vi "Main_Function_Motion Control.vi"(7 "Motion_Action":T3, 8 "Error In":errorcluster, 10 "Paremeter":T1={"Scan speed"=1, "Power"=0, "Angle"=0.0, "X"=0, "X"=0, "Xc"=0} {"Power" items=["Abs"=2, "Rel"=3]; "Scan speed" items=["X"=1, "Y"=2, "Z"=3, "Rotation"=4]}, 11 "VISA In":refnum<visa-resource-name>) -> (0 "Error Out":errorcluster, 2 "Response":string, 3 "VISA Out":refnum<visa-resource-name>)   [LabVIEW 2015]
uses:
  Control/Control_Motion Action.ctl
  Control/Control_Axis Number.ctl
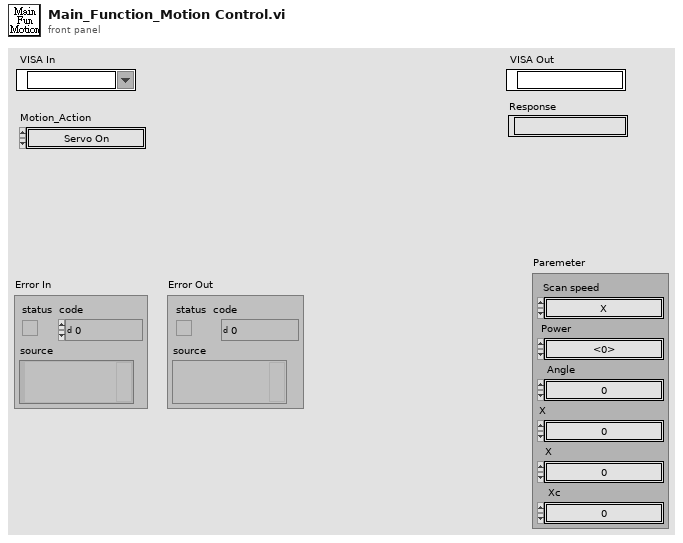
[diagram p1: front panel]
types:
  T1 = typedef "Control_手動測試_軸參數.ctl" = cluster{"Scan speed":T2, "Power":u16, "Angle":dbl, "X":i32, "X":i32, "Xc":i32}
  T2 = typedef "Control_Axis Number.ctl" = u16
  T3 = typedef "Control_Motion Action.ctl" = enum16{"Servo On", "Servo Off", "Homing", "Set Position", "Set Speed", "Set Acc", "Set Deacc", "Start Move", "Read Status", "Read Position"}
  T4 = enum16{"Open Connect", "Write and Read", "Close Connect"}
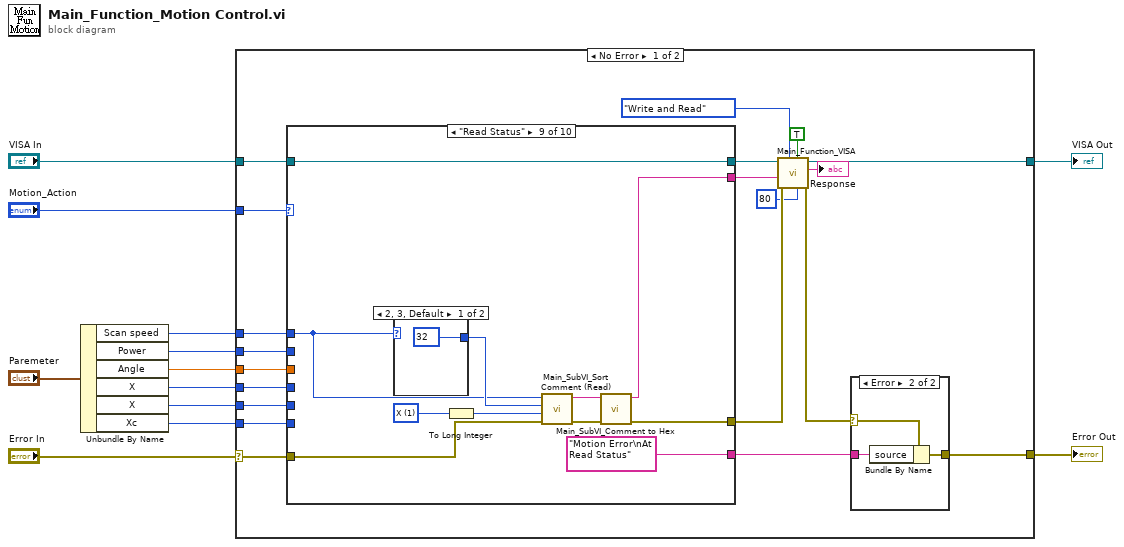
[diagram p0: block diagram]
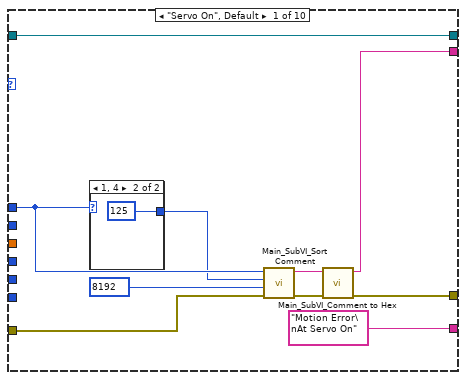
[diagram p3: hidden frame]
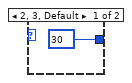
[diagram p4: hidden frame]
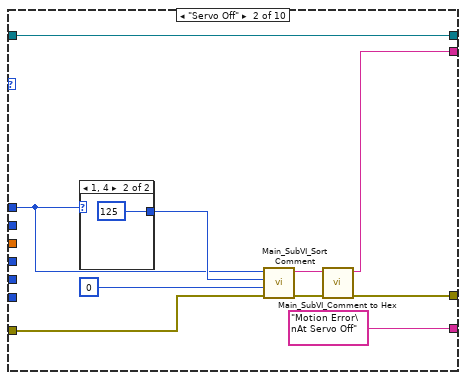
[diagram p5: hidden frame]
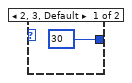
[diagram p6: hidden frame]
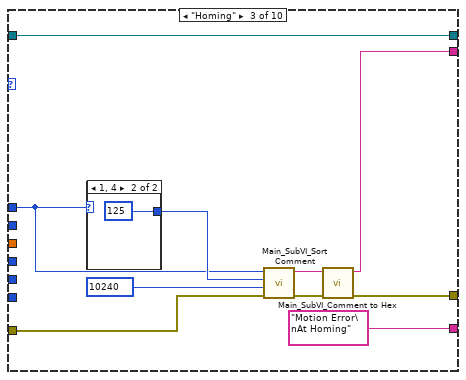
[diagram p7: hidden frame]
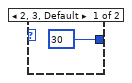
[diagram p8: hidden frame]
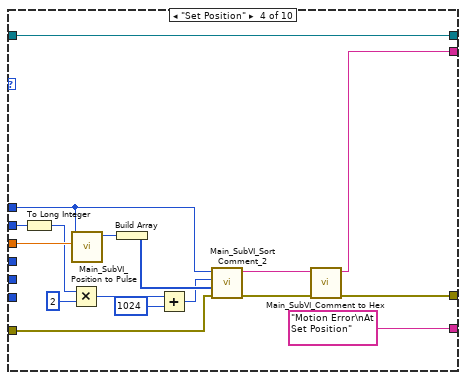
[diagram p9: hidden frame]
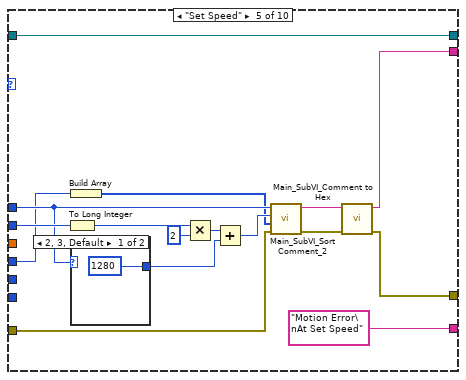
[diagram p10: hidden frame]
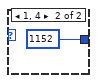
[diagram p11: hidden frame]
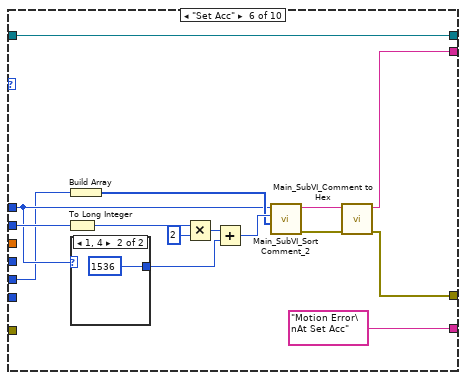
[diagram p12: hidden frame]
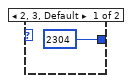
[diagram p13: hidden frame]
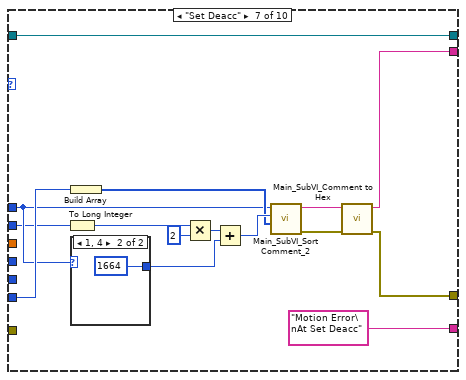
[diagram p14: hidden frame]
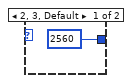
[diagram p15: hidden frame]
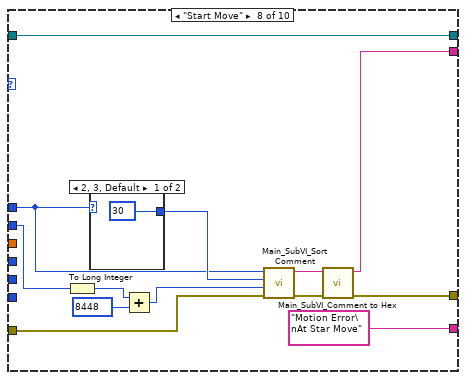
[diagram p16: hidden frame]
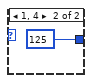
[diagram p17: hidden frame]
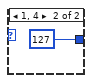
[diagram p18: hidden frame]
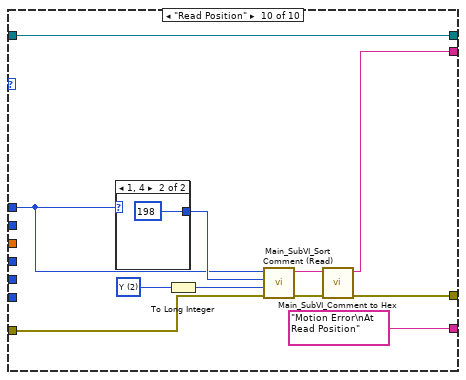
[diagram p19: hidden frame]
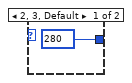
[diagram p20: hidden frame]
diagram:
  n1 = Unbundle By Name("Paremeter") -> ("Scan speed"=w6:T2, "Power"=w4:u16, "Angle"=w5:dbl, "X"=w3:i32, "X"=w2:i32, "Xc"=w1:i32)
  n2 = case shown="No Error" "Error In" {
    selector: "Error In" -> [w30 w184]
    tunnel: "Motion_Action" -> [w32 _]
    tunnel: w6 -> [w31 _]
    tunnel: "VISA In" -> [w29 w183]
    tunnel: [w26 w183] -> w8
    tunnel: [w22 w184] -> w9
    tunnel: w5 -> [w20 _]
    tunnel: w4 -> [w19 _]
    tunnel: w3 -> [w17 _]
    tunnel: w2 -> [w16 _]
    tunnel: w1 -> [w15 _]
    frame No Error {
      n3 = case shown="\"Read Status\"" w32 {
        tunnel: w31 -> [w45 w52 w65 w80 w98 w109 w126 w146 w162 w170]
        tunnel: w30 -> [w42 w53 w63 w78 w90 _ _ w148 w161 w171]
        tunnel: w29 -> [w40 w58 w62 w87 w93 w113 w128 w154 w158 w175]
        tunnel: [w40 w58 w62 w87 w93 w113 w128 w154 w158 w175] -> w28
        tunnel: [w39 w51 w61 w73 w94 w112 w129 w147 w166 w174] -> w27
        tunnel: ["Motion Error\nAt Servo On" ("source") "Motion Error\nAt Servo Off" ("source") "Motion Error\nAt Homing" ("source") "Motion Error\nAt Set Position" ("source") "Motion Error\nAt Set Speed" ("source") "Motion Error\nAt Set Acc" ("source") "Motion Error\nAt Set Deacc" ("source") "Motion Error\nAt Star Move" ("source") "Motion Error\nAt Read Status" ("source") "Motion Error\nAt Read Position" ("source")] -> w25
        tunnel: [w37 w49 w67 w74 w91 w111 w130 w150 w167 w173] -> w24
        tunnel: w20 -> [_ _ _ w83 _ _ _ _ _ _]
        tunnel: w19 -> [_ _ _ w82 w101 w110 w125 w142 _ _]
        tunnel: w17 -> [_ _ _ _ w97 _ _ _ _ _]
        tunnel: w16 -> [_ _ _ _ _ w108 _ _ _ _]
        tunnel: w15 -> [_ _ _ _ _ _ w127 _ _ _]
        frame "Servo On", Default {
          n4 = case shown="1, 4" w45 {
            tunnel: [30 ("t") 125 ("f")] -> w44
            frame 2, 3, Default {
            }
            frame 1, 4 {
            }
          }
          n5 = call "Main_SubVI_Sort Comment.vi"("Error In"=w42, "Data"=8192 ("t"), "Register  Address"=w44, "Axis Number"=w45) -> ("Error Out"=w41:errorcluster, "Command"=w43:string)  [unwired: 6 in]
          n6 = call "Main_SubVI_Comment to Hex.vi"("Error In"=w41, "Normal In"=w43) -> ("Error Out"=w37:errorcluster, "Hex Out"=w39:string)  [unwired: 8 in]
        }
        frame "Servo Off" {
          n7 = case shown="1, 4" w52 {
            tunnel: [30 ("t") 125 ("f")] -> w56
            frame 2, 3, Default {
            }
            frame 1, 4 {
            }
          }
          n8 = call "Main_SubVI_Sort Comment.vi"("Error In"=w53, "Data"=0 ("t"), "Register  Address"=w56, "Axis Number"=w52) -> ("Error Out"=w54:errorcluster, "Command"=w55:string)  [unwired: 6 in]
          n9 = call "Main_SubVI_Comment to Hex.vi"("Error In"=w54, "Normal In"=w55) -> ("Error Out"=w49:errorcluster, "Hex Out"=w51:string)  [unwired: 8 in]
        }
        frame "Homing" {
          n10 = case shown="1, 4" w65 {
            tunnel: [30 ("t") 125 ("f")] -> w66
            frame 2, 3, Default {
            }
            frame 1, 4 {
            }
          }
          n11 = call "Main_SubVI_Sort Comment.vi"("Error In"=w63, "Data"=10240, "Register  Address"=w66, "Axis Number"=w65) -> ("Error Out"=w69:errorcluster, "Command"=w70:string)  [unwired: 6 in]
          n12 = call "Main_SubVI_Comment to Hex.vi"("Error In"=w69, "Normal In"=w70) -> ("Error Out"=w67:errorcluster, "Hex Out"=w61:string)  [unwired: 8 in]
        }
        frame "Set Position" {
          n13 = To Long Integer(number=w82) -> (32bit integer=w81:i32)
          n14 = Multiply(x=w81, y=2) -> (x*y=w85:i32)
          n15 = call "Main_SubVI_Position to Pulse.vi"("Postion"=w83, "Axis Number"=w80) -> ("Pulse"=w89:i32)  [unwired: 8 in, 1 out]
          n16 = Build Array(w89) -> (w88:i32[])
          n17 = Add(x=w85, y=1024) -> (x+y=w79:i32)
          n18 = call "Main_SubVI_Sort Comment_2.vi"("Error In"=w78, "Datas"=w88, "Register  Address"=w79, "Axis Number"=w80) -> ("Error Out"=w75:errorcluster, "Command"=w76:string)  [unwired: 6 in]
          n19 = call "Main_SubVI_Comment to Hex.vi"("Error In"=w75, "Normal In"=w76) -> ("Error Out"=w74:errorcluster, "Hex Out"=w73:string)  [unwired: 8 in]
        }
        frame "Set Speed" {
          n20 = To Long Integer(number=w101) -> (32bit integer=w100:i32)
          n21 = Build Array(w97) -> (w96:i32[])
          n22 = case shown="2, 3, Default" w98 {
            tunnel: [1280 ("t") 1152 ("f")] -> w102
            frame 2, 3, Default {
            }
            frame 1, 4 {
            }
          }
          n23 = Multiply(x=w100, y=2) -> (x*y=w104:i32)
          n24 = Add(x=w104, y=w102) -> (x+y=w99:i32)
          n25 = call "Main_SubVI_Sort Comment_2.vi"("Error In"=w90, "Datas"=w96, "Register  Address"=w99, "Axis Number"=w98) -> ("Error Out"=w92:errorcluster, "Command"=w95:string)  [unwired: 6 in]
          n26 = call "Main_SubVI_Comment to Hex.vi"("Error In"=w92, "Normal In"=w95) -> ("Error Out"=w91:errorcluster, "Hex Out"=w94:string)  [unwired: 8 in]
        }
        frame "Set Acc" {
          n27 = To Long Integer(number=w110) -> (32bit integer=w118:i32)
          n28 = Build Array(w108) -> (w116:i32[])
          n29 = case shown="1, 4" w109 {
            tunnel: [2304 ("t") 1536 ("f")] -> w119
            frame 2, 3, Default {
            }
            frame 1, 4 {
            }
          }
          n30 = Multiply(x=w118, y=2) -> (x*y=w121:i32)
          n31 = Add(x=w121, y=w119) -> (x+y=w117:i32)
          n32 = call "Main_SubVI_Sort Comment_2.vi"("Datas"=w116, "Register  Address"=w117, "Axis Number"=w109) -> ("Error Out"=w114:errorcluster, "Command"=w115:string)  [unwired: 7 in]
          n33 = call "Main_SubVI_Comment to Hex.vi"("Error In"=w114, "Normal In"=w115) -> ("Error Out"=w111:errorcluster, "Hex Out"=w112:string)  [unwired: 8 in]
        }
        frame "Set Deacc" {
          n34 = To Long Integer(number=w125) -> (32bit integer=w136:i32)
          n35 = Build Array(w127) -> (w134:i32[])
          n36 = case shown="1, 4" w126 {
            tunnel: [2560 ("t") 1664 ("f")] -> w137
            frame 2, 3, Default {
            }
            frame 1, 4 {
            }
          }
          n37 = Multiply(x=w136, y=2) -> (x*y=w139:i32)
          n38 = Add(x=w139, y=w137) -> (x+y=w135:i32)
          n39 = call "Main_SubVI_Sort Comment_2.vi"("Datas"=w134, "Register  Address"=w135, "Axis Number"=w126) -> ("Error Out"=w132:errorcluster, "Command"=w133:string)  [unwired: 7 in]
          n40 = call "Main_SubVI_Comment to Hex.vi"("Error In"=w132, "Normal In"=w133) -> ("Error Out"=w130:errorcluster, "Hex Out"=w129:string)  [unwired: 8 in]
        }
        frame "Start Move" {
          n41 = To Long Integer(number=w142) -> (32bit integer=w144:i32)
          n42 = case shown="2, 3, Default" w146 {
            tunnel: [30 ("t") 125 ("f")] -> w153
            frame 2, 3, Default {
            }
            frame 1, 4 {
            }
          }
          n43 = Add(x=w144, y=8448) -> (x+y=w143:i32)
          n44 = call "Main_SubVI_Sort Comment.vi"("Error In"=w148, "Data"=w143, "Register  Address"=w153, "Axis Number"=w146) -> ("Error Out"=w151:errorcluster, "Command"=w152:string)  [unwired: 6 in]
          n45 = call "Main_SubVI_Comment to Hex.vi"("Error In"=w151, "Normal In"=w152) -> ("Error Out"=w150:errorcluster, "Hex Out"=w147:string)  [unwired: 8 in]
        }
        frame "Read Status" {
          w160 = T2 1 items=["X"=1, "Y"=2, "Z"=3, "Rotation"=4] ("Axis Number")
          n46 = case shown="2, 3, Default" w162 {
            tunnel: [32 ("f") 127 ("t")] -> w163
            frame 2, 3, Default {
            }
            frame 1, 4 {
            }
          }
          n47 = To Long Integer(number=w160) -> (32bit integer=w159:i32)
          n48 = call "Main_SubVI_Sort Comment (Read).vi"("Error In"=w161, "Number"=w159, "Register  Address"=w163, "Axis Number"=w162) -> ("Error Out"=w164:errorcluster, "Command"=w165:string)  [unwired: 6 in]
          n49 = call "Main_SubVI_Comment to Hex.vi"("Error In"=w164, "Normal In"=w165) -> ("Error Out"=w167:errorcluster, "Hex Out"=w166:string)  [unwired: 8 in]
        }
        frame "Read Position" {
          w177 = T2 2 items=["X"=1, "Y"=2, "Z"=3, "Rotation"=4] ("Axis Number")
          n50 = case shown="1, 4" w170 {
            tunnel: [280 ("f") 198 ("t")] -> w178
            frame 2, 3, Default {
            }
            frame 1, 4 {
            }
          }
          n51 = To Long Integer(number=w177) -> (32bit integer=w176:i32)
          n52 = call "Main_SubVI_Sort Comment (Read).vi"("Error In"=w171, "Number"=w176, "Register  Address"=w178, "Axis Number"=w170) -> ("Error Out"=w179:errorcluster, "Command"=w180:string)  [unwired: 6 in]
          n53 = call "Main_SubVI_Comment to Hex.vi"("Error In"=w179, "Normal In"=w180) -> ("Error Out"=w173:errorcluster, "Hex Out"=w174:string)  [unwired: 8 in]
        }
      }
      n54 = call "Main_Function_VISA.vi"("Delay Time"=u32 80, "CRC"=TRUE, "Action_VISA"=T4."Write and Read", "Error In"=w24, "Comment"=w27, "VISA In"=w28) -> ("Error Out"=w23:errorcluster, "Response"=→"Response":string, "VISA Out"=w26:refnum<visa-resource-name>)  [unwired: 3 in]
      n55 = case shown="Error" w23 {
        selector: w23 -> [w33 w36]
        tunnel: [w33 w35] -> w22
        tunnel: w25 -> [_ w34]
        frame No Error {
        }
        frame Error {
          n56 = Bundle By Name(cluster=w36, "source"=w34) -> (w35:errorcluster)
        }
      }
    }
    frame Error {
    }
  }
  "Error Out" <- w9
  "VISA Out" <- w8
